vi "stopStartMotionAcq.vi"(0 "error out":errorcluster, 3 "timeout":i32, 5 "notifier out":refnum<notifier>, 6 "frameFilenameArray":path[](array[path]), 7 "z inc (mm)":dbl, 8 "zIdx":i32, 9 "System no.":i32, 10 "sCMOShandle":u32) -> (4 "Stopped":bool)   [LabVIEW 2015]
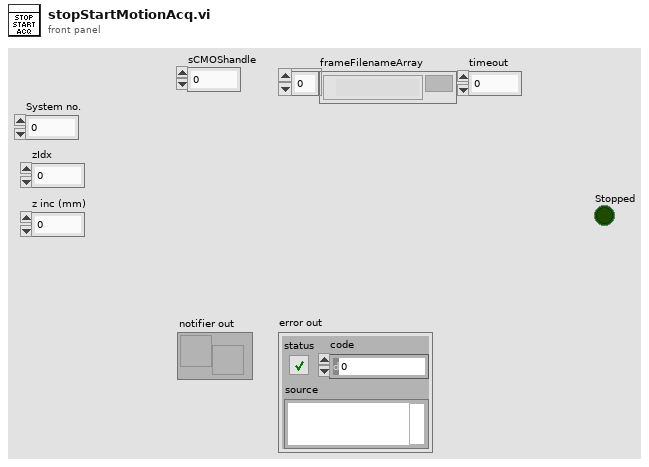
[diagram p1: front panel]
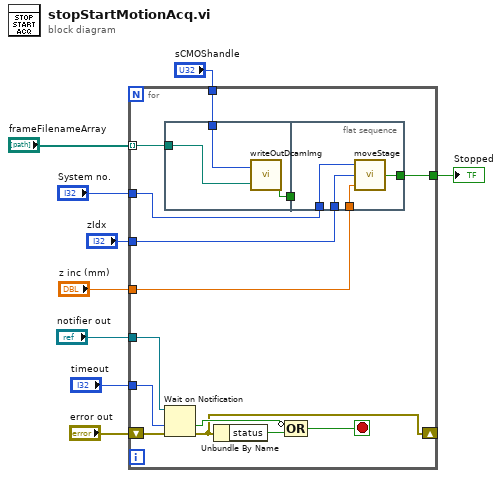
[diagram p0: block diagram]
diagram:
  n1 = for {
    tunnel: "notifier out" -> [w23]
    shift-right: [w20] -> _
    shift-left: "error out" -> [w22]
    tunnel: "timeout" -> [w18]
    tunnel: "z inc (mm)" -> [w17]
    tunnel: "frameFilenameArray" -> [w15] mode=indexing
    tunnel: "System no." -> [w14]
    tunnel: "zIdx" -> [w13]
    tunnel: [w11] -> w2
    tunnel: "sCMOShandle" -> [w10]
    stop <- w16 stop-if-true
    n2 = flat-sequence {
      tunnel: w15 -> [w26]
      tunnel: [w25] -> w12
      tunnel: w10 -> [w24]
      tunnel: w17 -> [w30]
      tunnel: [w29] -> w11
      tunnel: w12 -> [_]
      tunnel: w14 -> [w28]
      tunnel: w13 -> [w27]
      frame #0 {
        n3 = call "writeOutDcamImg.vi"("stackFname"=w26, "sCMOShandle"=w24) -> ("stackComplete"=w25:bool)
      }
      frame #1 {
        n4 = call "moveStage.vi"("inc (mm)"=w30, "axisIdx"=w27, "System no."=w28) -> ("Stopped"=w29:bool)
      }
    }
    n5 = Wait on Notification(notifier=w23, timeout in ms (-1)=w18, error in (no error)=w22) -> (timed out?=w21:bool, error out=w20:errorcluster)  [unwired: 1 in, 2 out]
    n6 = Unbundle By Name(w20) -> ("status"=w19:bool)
    n7 = Compound Arithmetic op=OR(invert w21, w19) -> (w16:bool)
  }
  "Stopped" <- w2
